vi "실습 8-3.vi"() -> ()   [LabVIEW 2014]
panel:
  in  "경로":path
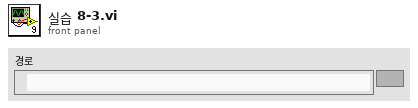
[diagram p1: front panel]
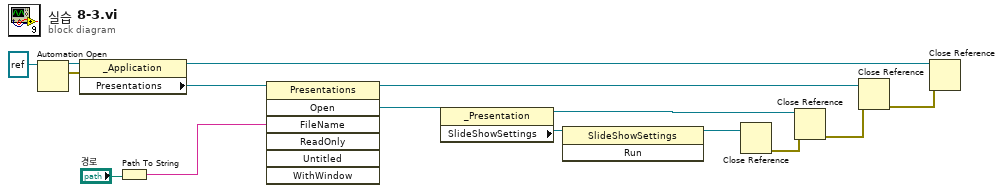
[diagram p0: block diagram]
diagram:
  n1 = Automation Open(Automation Refnum=refnum<k7> refnum ("PowerPoint._Application")) -> (Automation Refnum=w14:refnum<k7>, error out=w13:errorcluster)  [unwired: 3 in]
  n2 = property class="_Application"(reference=w14, error in=w13) -> (reference out=w4:refnum<k7>, "Presentations"=w12:refnum<k7>)  [unwired: 1 out]
  n3 = Path To String(path="경로") -> (string=w10:string)
  n4 = invoke class="Presentations" method="Open"(reference=w12, "FileName"=w10) -> (reference out=w5:refnum<k7>, "Open"=w9:refnum<k7>)  [unwired: 5 in, 5 out]
  n5 = property class="_Presentation"(reference=w9) -> (reference out=w6:refnum<k7>, "SlideShowSettings"=w8:refnum<k7>)  [unwired: 1 in, 1 out]
  n6 = invoke class="SlideShowSettings" method="Run"(reference=w8) -> (reference out=w7:refnum<k7>)  [unwired: 2 in, 2 out]
  n7 = Close Reference(reference=w7) -> (error out=w3:errorcluster)  [unwired: 1 in]
  n8 = Close Reference(reference=w6, error in (no error)=w3) -> (error out=w2:errorcluster)
  n9 = Close Reference(reference=w5, error in (no error)=w2) -> (error out=w1:errorcluster)
  n10 = Close Reference(reference=w4, error in (no error)=w1) -> ()  [unwired: 1 out]
